vi "NI6602.ProcCases.vi"(0 "i ref in":refnum<vi>, 1 "selector":string, 2 "Data":T1, 3 "call cluster":T2={"Object"="", "Selector"="", "CallType"=enum."synchronous", "Async Object"="", "Async Selector"="", "Data Descriptor"="", "Data"=[], "Error #"=0, "Expire"=0}, 5 "error in (no error)":errorcluster) -> (14 "i ref out":refnum<vi>, 17 "answer cluster":T2={"Object"="", "Selector"="", "CallType"=enum."synchronous", "Async Object"="", "Async Selector"="", "Data Descriptor"="", "Data"=[], "Error #"=0, "Expire"=0}, 19 "error out":errorcluster)   [LabVIEW 2014, in "NI6602.lvlib"]
doc: "This method is called by a process from within the default case in the event loop. The methods of a class that are linked to events will be called from THIS method. Add your code here."
uses:
  NI6602.lvlib
  CS_Core/BaseProcess/BaseProcess.lvlib
  CS_Core/CSApplicationBaseClasses/DeviceBase/DeviceBase.lvlib
  CS_Core/CSSystem/CoreLib/CoreLib.string 2 byte array.vi
  CS_Core/CSSystem/CoreLib/CoreLib.lvlib
  CSlibraries-extern/DimLVEvent/LVDimInterface/LVDimInterface.lvlib
  CS_Core/CSSystem/CoreLib/CoreLib.byte array 2 double.vi
  CS_Core/CSSystem/CoreDefs/CoreDefs.call_type.ctl
  CS_Core/CSSystem/CoreDefs/CoreDefs.rawDataType.ctl
  CS_Core/BaseProcess/BaseProcess.descriptor string definition.ctl
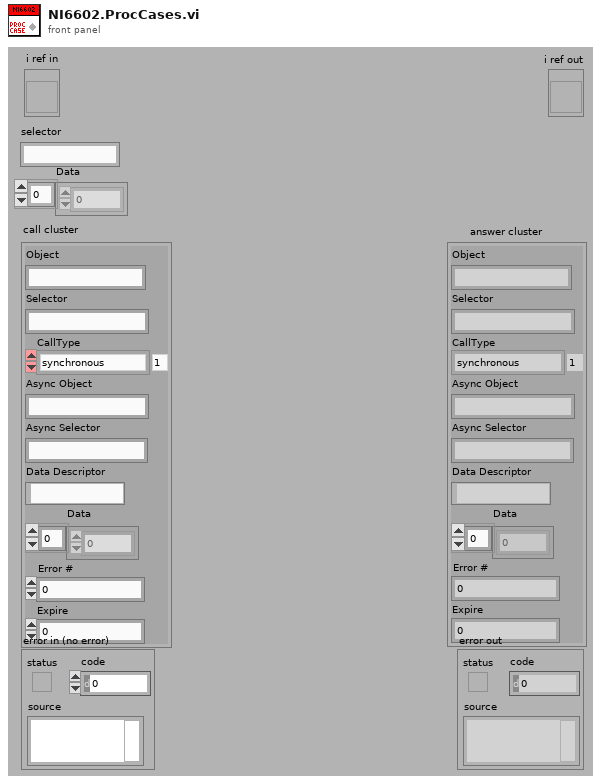
[diagram p1: front panel]
types:
  T1 = typedef "CoreDefs.rawDataType.ctl" = i8[]
  T2 = typedef "CoreDefs.call_type.ctl" = cluster{"Object":string, "Selector":string, "CallType":enum16{"simple", "synchronous", "asynchronous"}, "Async Object":string, "Async Selector":string, "Data Descriptor":T3, "Data":T1, "Error #":i32, "Expire":u32}
  T3 = typedef "BaseProcess.lvlib/BaseProcess.descriptor string definition.ctl" = string
  T4 = typedef "NI6602.lvlib/NI6602.i attribute.ctl" = cluster{"CounterDAQ Channels":cluster{"task":refnum<k21>, "Channel Name":string}[], "RateServiceIDs":i32[], "Running?":bool, "IntegralServiceIDs":i32[], "ThresholdID":i32, "Threshold":dbl, "IntegralValues":dbl[], "Stopped?":bool}
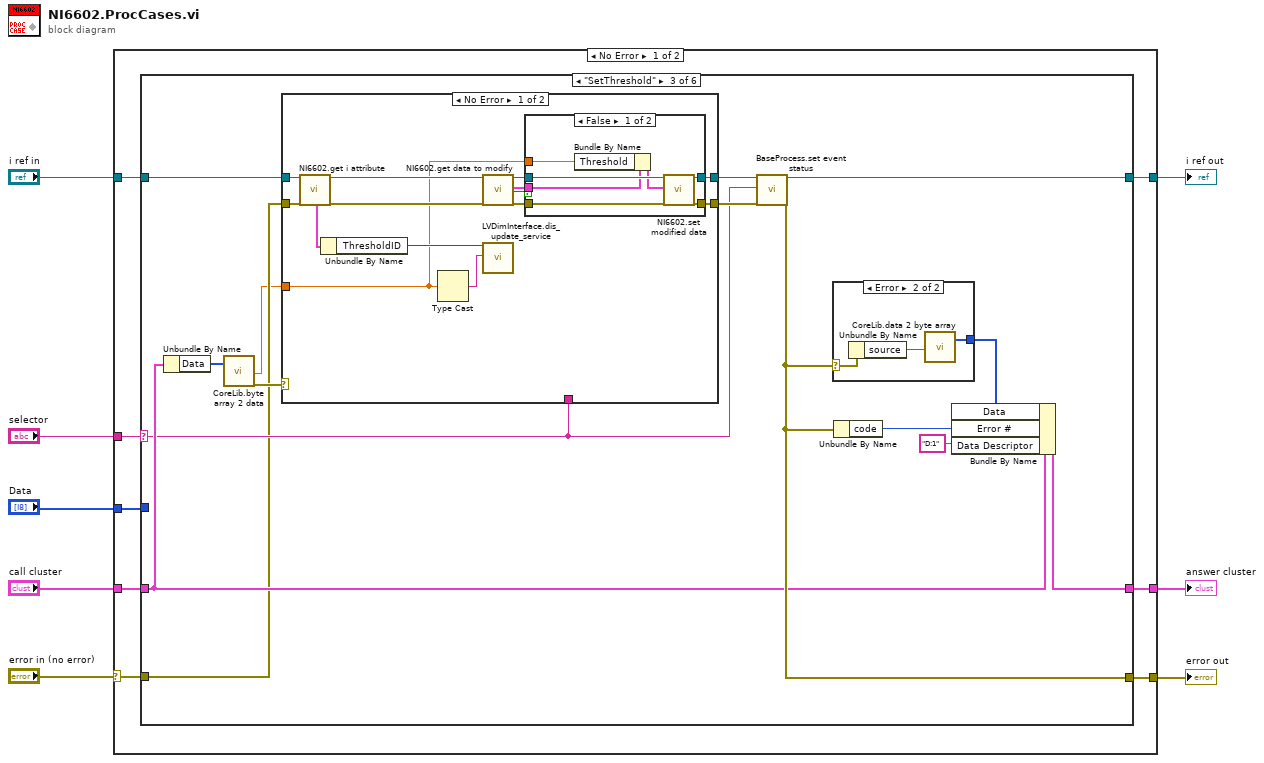
[diagram p0: block diagram]
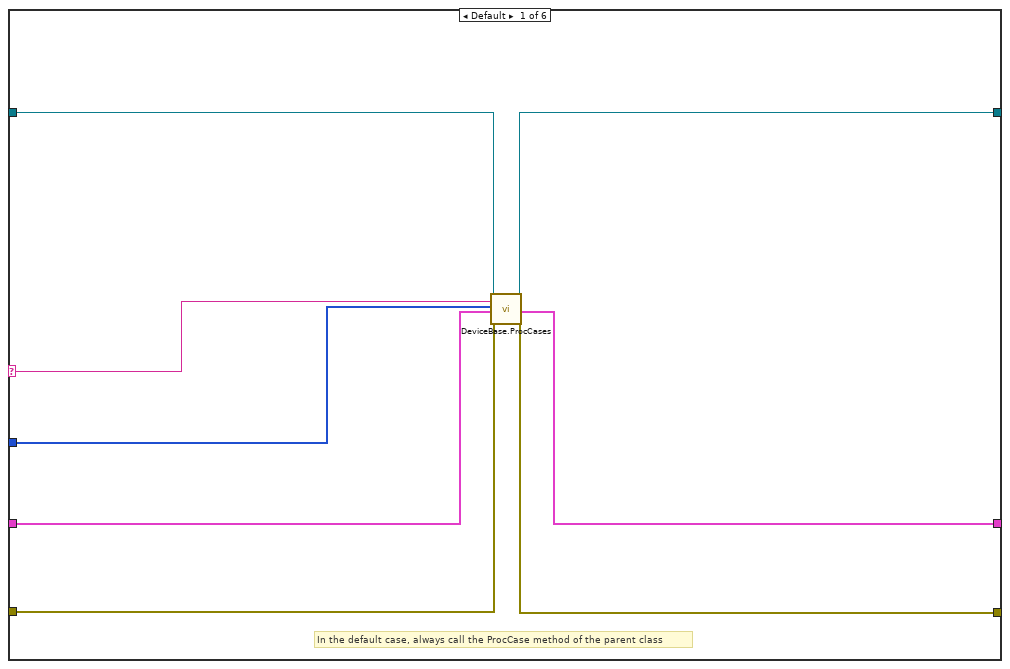
[diagram p2: hidden frame]
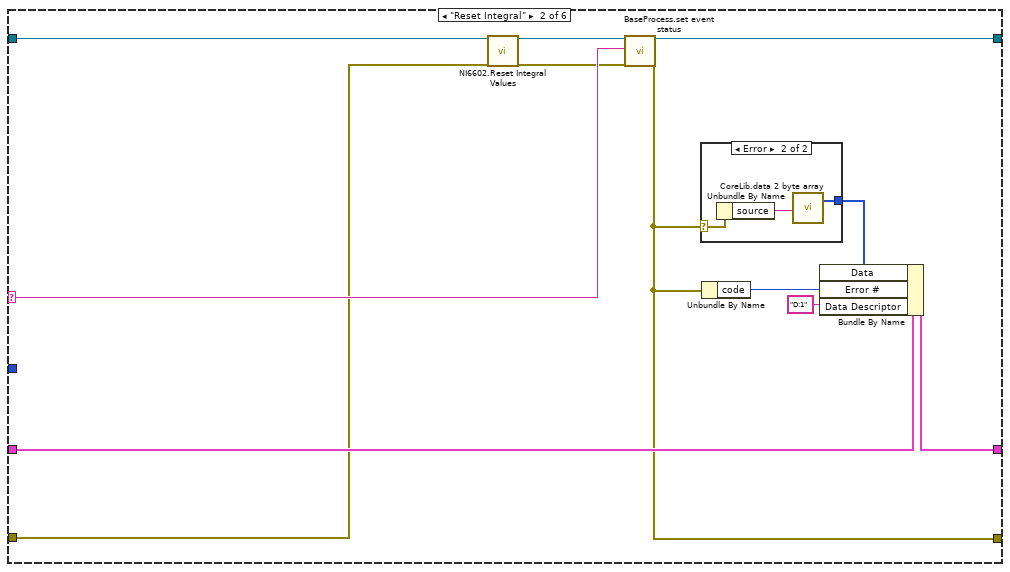
[diagram p3: hidden frame]
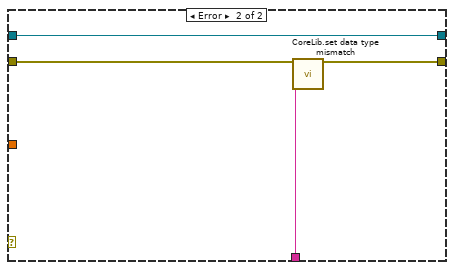
[diagram p6: hidden frame]
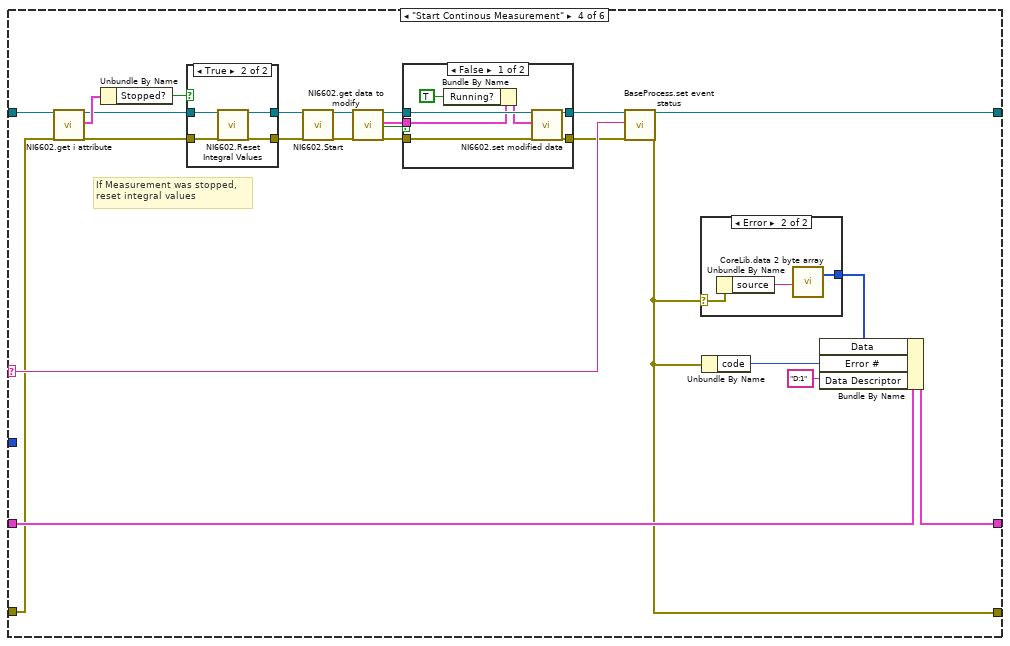
[diagram p8: hidden frame]
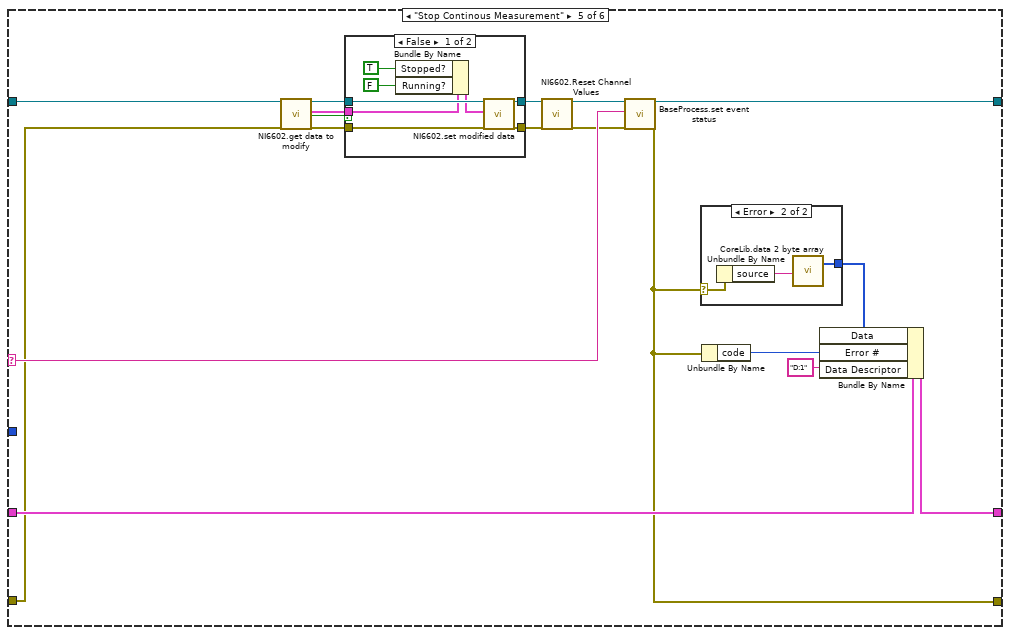
[diagram p12: hidden frame]
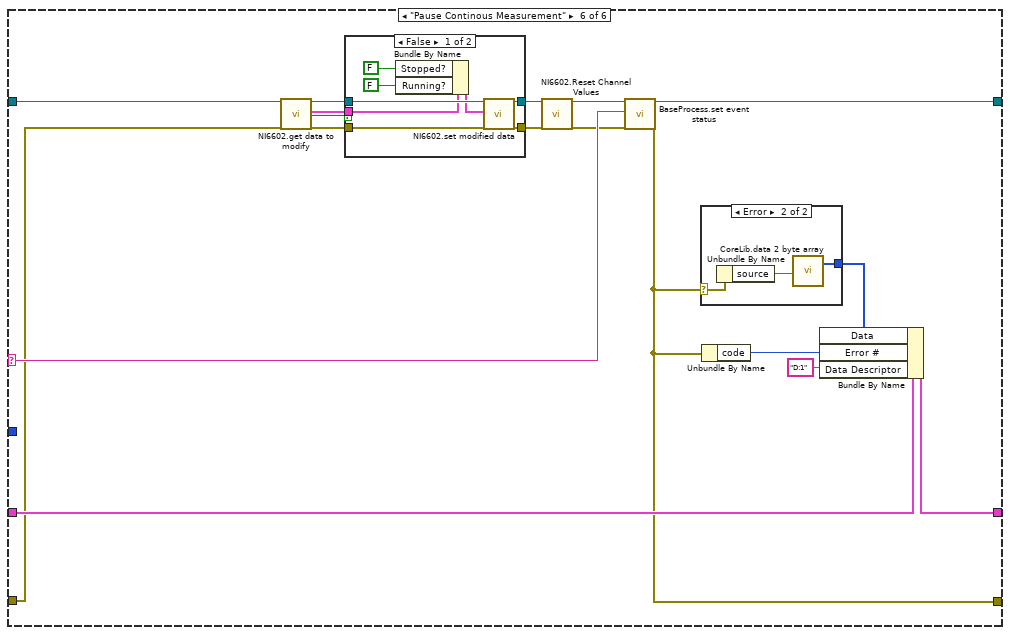
[diagram p15: hidden frame]
diagram:
  n1 = case shown="No Error" "error in (no error)" {
    selector: "error in (no error)" -> [w9 w189]
    tunnel: "selector" -> [w16 _]
    tunnel: [w15 w190] -> w7
    tunnel: "Data" -> [w14 _]
    tunnel: "call cluster" -> [w13 w190]
    tunnel: "i ref in" -> [w12 w191]
    tunnel: [w11 w191] -> w3
    tunnel: [w10 w189] -> w2
    frame No Error {
      n2 = case shown="\"SetThreshold\"" w16 {
        selector: w16 -> [w19 w31 w43 w103 w139 w170]
        tunnel: w14 -> [w17 _ _ _ _ _]
        tunnel: w12 -> [w18 w28 w40 w91 w131 w162]
        tunnel: [w24 w30 w50 w102 w138 w169] -> w11
        tunnel: w13 -> [w20 w35 w45 w107 w143 w174]
        tunnel: [w21 w34 w53 w106 w142 w173] -> w15
        tunnel: w9 -> [w23 w25 w42 w92 w132 w163]
        tunnel: [w22 w32 w51 w104 w140 w171] -> w10
        frame Default {
          # "In the default case, always call the ProcCase method of the parent class"
          n3 = call "DeviceBase.ProcCases.vi"("i ref in"=w18, "selector"=w19, "Data"=w17, "call cluster"=w20, "error in (no error)"=w23) -> ("i ref out"=w24:refnum<vi>, "answer cluster"=w21:T2, "error out"=w22:errorcluster)  [unwired: 12 in]
        }
        frame "Reset Integral" {
          n4 = call "NI6602.Reset Integral Values.vi"("i ref in"=w28, "error in (no error)"=w25) -> ("i ref out"=w27:refnum<vi>, "error out"=w26:errorcluster)  [unwired: 16 in]
          n5 = call "BaseProcess.set event status.vi"("i ref in"=w27, "EventStatus"=w31, "error in (no error)"=w26) -> ("i ref out"=w30:refnum<vi>, "error out"=w32:errorcluster)  [unwired: 14 in, 1 out]
          n6 = case shown="Error" w32 {
            selector: w32 -> [_ w39]
            tunnel: [_ w38] -> w33
            frame No Error {
            }
            frame Error {
              n7 = Unbundle By Name(w39) -> ("source"=w37:string)
              n8 = call-poly "CoreLib.data 2 byte array.vi"("string"=w37) -> ("byteArray out"=w38:T1)  [unwired: 18 in]
            }
          }
          n9 = Unbundle By Name(w32) -> ("code"=w36:i32)
          n10 = Bundle By Name(cluster=w35, "Data"=w33, "Error #"=w36, "Data Descriptor"="D:1") -> (w34:T2)
        }
        frame "SetThreshold" {
          n11 = Unbundle By Name(w45) -> ("Data"=w46:T1)
          n12 = call-poly "CoreLib.byte array 2 data.vi"("byteArray"=w46) -> ("d64"=w41:dbl, "error out"=w44:errorcluster)  [unwired: 16 in, 1 out]
          n13 = case shown="No Error" w44 {
            tunnel: [w64 w78] -> w48
            tunnel: [w63 w81] -> w47
            tunnel: w43 -> [_ w80]
            tunnel: w42 -> [w61 w79]
            tunnel: w41 -> [w55 _]
            tunnel: w40 -> [w60 w78]
            frame No Error {
              n14 = call "NI6602.get i attribute.vi"("i ref in"=w60, "error in (no error)"=w61) -> ("i ref out"=w59:refnum<vi>, "i attribute"=w58:T4, "error out"=w62:errorcluster)  [unwired: 15 in]
              n15 = Unbundle By Name(w58) -> ("ThresholdID"=w57:i32)
              n16 = Type Cast(x=w55) -> (*(type *) &x=w56:string)  [unwired: 1 in]
              n17 = call "NI6602.get data to modify.vi"("i ref in"=w59, "error in (no error)"=w62) -> ("i ref out"=w66:refnum<vi>, "i attribute"=w68:T4, "timed out"=w67:bool, "error out"=w65:errorcluster)  [unwired: 14 in]
              n18 = call "LVDimInterface.dis_update_service.vi"("my_serviceID"=w57, "data"=w56) -> ()  [unwired: 15 in, 3 out]
              n19 = case shown="False" w67 {
                tunnel: w65 -> [w75 w76]
                tunnel: [w74 w76] -> w63
                tunnel: w66 -> [w73 w77]
                tunnel: [w72 w77] -> w64
                tunnel: w68 -> [w71 _]
                tunnel: w55 -> [w69 _]
                frame False {
                  n20 = Bundle By Name(cluster=w71, "Threshold"=w69) -> (w70:T4)
                  n21 = call "NI6602.set modified data.vi"("i ref in"=w73, "i attribute"=w70, "error in (no error)"=w75) -> ("i ref out"=w72:refnum<vi>, "error out"=w74:errorcluster)  [unwired: 15 in]
                }
                frame True {
                }
              }
            }
            frame Error {
              n22 = call "CoreLib.set data type mismatch.vi"("error in (no error)"=w79, "error source"=w80) -> ("error out"=w81:errorcluster)  [unwired: 17 in]
            }
          }
          n23 = call "BaseProcess.set event status.vi"("i ref in"=w48, "EventStatus"=w43, "error in (no error)"=w47) -> ("i ref out"=w50:refnum<vi>, "error out"=w51:errorcluster)  [unwired: 14 in, 1 out]
          n24 = case shown="Error" w51 {
            selector: w51 -> [_ w84]
            tunnel: [_ w83] -> w52
            frame No Error {
            }
            frame Error {
              n25 = Unbundle By Name(w84) -> ("source"=w82:string)
              n26 = call-poly "CoreLib.data 2 byte array.vi"("string"=w82) -> ("byteArray out"=w83:T1)  [unwired: 18 in]
            }
          }
          n27 = Unbundle By Name(w51) -> ("code"=w54:i32)
          n28 = Bundle By Name(cluster=w45, "Data"=w52, "Error #"=w54, "Data Descriptor"="D:1") -> (w53:T2)
        }
        frame "Start Continous Measurement" {
          # "If Measurement was stopped,\nreset integral values"
          n29 = call "NI6602.get i attribute.vi"("i ref in"=w91, "error in (no error)"=w92) -> ("i ref out"=w87:refnum<vi>, "i attribute"=w90:T4, "error out"=w88:errorcluster)  [unwired: 15 in]
          n30 = Unbundle By Name(w90) -> ("Stopped?"=w89:bool)
          n31 = case shown="True" w89 {
            tunnel: w88 -> [w109 w114]
            tunnel: w87 -> [w110 w113]
            tunnel: [w110 w112] -> w86
            tunnel: [w109 w111] -> w85
            frame False {
            }
            frame True {
              n32 = call "NI6602.Reset Integral Values.vi"("i ref in"=w113, "error in (no error)"=w114) -> ("i ref out"=w112:refnum<vi>, "error out"=w111:errorcluster)  [unwired: 16 in]
            }
          }
          n33 = call "NI6602.Start.vi"("i ref in"=w86, "error in (no error)"=w85) -> ("i ref out"=w93:refnum<vi>, "error out"=w94:errorcluster)  [unwired: 16 in]
          n34 = call "NI6602.get data to modify.vi"("i ref in"=w93, "error in (no error)"=w94) -> ("i ref out"=w98:refnum<vi>, "i attribute"=w100:T4, "timed out"=w99:bool, "error out"=w97:errorcluster)  [unwired: 14 in]
          n35 = case shown="False" w99 {
            tunnel: w97 -> [w121 w122]
            tunnel: [w120 w122] -> w95
            tunnel: w98 -> [w119 w123]
            tunnel: [w118 w123] -> w96
            tunnel: w100 -> [w117 _]
            frame False {
              n36 = Bundle By Name(cluster=w117, "Running?"=TRUE) -> (w116:T4)
              n37 = call "NI6602.set modified data.vi"("i ref in"=w119, "i attribute"=w116, "error in (no error)"=w121) -> ("i ref out"=w118:refnum<vi>, "error out"=w120:errorcluster)  [unwired: 15 in]
            }
            frame True {
            }
          }
          n38 = call "BaseProcess.set event status.vi"("i ref in"=w96, "EventStatus"=w103, "error in (no error)"=w95) -> ("i ref out"=w102:refnum<vi>, "error out"=w104:errorcluster)  [unwired: 14 in, 1 out]
          n39 = case shown="Error" w104 {
            selector: w104 -> [_ w126]
            tunnel: [_ w125] -> w105
            frame No Error {
            }
            frame Error {
              n40 = Unbundle By Name(w126) -> ("source"=w124:string)
              n41 = call-poly "CoreLib.data 2 byte array.vi"("string"=w124) -> ("byteArray out"=w125:T1)  [unwired: 18 in]
            }
          }
          n42 = Unbundle By Name(w104) -> ("code"=w108:i32)
          n43 = Bundle By Name(cluster=w107, "Data"=w105, "Error #"=w108, "Data Descriptor"="D:1") -> (w106:T2)
        }
        frame "Stop Continous Measurement" {
          n44 = call "NI6602.get data to modify.vi"("i ref in"=w131, "error in (no error)"=w132) -> ("i ref out"=w134:refnum<vi>, "i attribute"=w136:T4, "timed out"=w135:bool, "error out"=w133:errorcluster)  [unwired: 14 in]
          n45 = case shown="False" w135 {
            tunnel: w133 -> [w152 w153]
            tunnel: [w151 w153] -> w130
            tunnel: w134 -> [w150 w154]
            tunnel: [w149 w154] -> w129
            tunnel: w136 -> [w148 _]
            frame False {
              n46 = Bundle By Name(cluster=w148, "Stopped?"=TRUE, "Running?"=FALSE) -> (w147:T4)
              n47 = call "NI6602.set modified data.vi"("i ref in"=w150, "i attribute"=w147, "error in (no error)"=w152) -> ("i ref out"=w149:refnum<vi>, "error out"=w151:errorcluster)  [unwired: 15 in]
            }
            frame True {
            }
          }
          n48 = call "NI6602.Reset Channel Values.vi"("i ref in"=w129, "error in (no error)"=w130) -> ("i ref out"=w127:refnum<vi>, "error out"=w128:errorcluster)  [unwired: 16 in]
          n49 = call "BaseProcess.set event status.vi"("i ref in"=w127, "EventStatus"=w139, "error in (no error)"=w128) -> ("i ref out"=w138:refnum<vi>, "error out"=w140:errorcluster)  [unwired: 14 in, 1 out]
          n50 = case shown="Error" w140 {
            selector: w140 -> [_ w157]
            tunnel: [_ w156] -> w141
            frame No Error {
            }
            frame Error {
              n51 = Unbundle By Name(w157) -> ("source"=w155:string)
              n52 = call-poly "CoreLib.data 2 byte array.vi"("string"=w155) -> ("byteArray out"=w156:T1)  [unwired: 18 in]
            }
          }
          n53 = Unbundle By Name(w140) -> ("code"=w144:i32)
          n54 = Bundle By Name(cluster=w143, "Data"=w141, "Error #"=w144, "Data Descriptor"="D:1") -> (w142:T2)
        }
        frame "Pause Continous Measurement" {
          n55 = call "NI6602.get data to modify.vi"("i ref in"=w162, "error in (no error)"=w163) -> ("i ref out"=w165:refnum<vi>, "i attribute"=w167:T4, "timed out"=w166:bool, "error out"=w164:errorcluster)  [unwired: 14 in]
          n56 = case shown="False" w166 {
            tunnel: w164 -> [w183 w184]
            tunnel: [w182 w184] -> w161
            tunnel: w165 -> [w181 w185]
            tunnel: [w180 w185] -> w160
            tunnel: w167 -> [w179 _]
            frame False {
              n57 = Bundle By Name(cluster=w179, "Stopped?"=FALSE, "Running?"=FALSE) -> (w178:T4)
              n58 = call "NI6602.set modified data.vi"("i ref in"=w181, "i attribute"=w178, "error in (no error)"=w183) -> ("i ref out"=w180:refnum<vi>, "error out"=w182:errorcluster)  [unwired: 15 in]
            }
            frame True {
            }
          }
          n59 = call "NI6602.Reset Channel Values.vi"("i ref in"=w160, "error in (no error)"=w161) -> ("i ref out"=w158:refnum<vi>, "error out"=w159:errorcluster)  [unwired: 16 in]
          n60 = call "BaseProcess.set event status.vi"("i ref in"=w158, "EventStatus"=w170, "error in (no error)"=w159) -> ("i ref out"=w169:refnum<vi>, "error out"=w171:errorcluster)  [unwired: 14 in, 1 out]
          n61 = case shown="Error" w171 {
            selector: w171 -> [_ w188]
            tunnel: [_ w187] -> w172
            frame No Error {
            }
            frame Error {
              n62 = Unbundle By Name(w188) -> ("source"=w186:string)
              n63 = call-poly "CoreLib.data 2 byte array.vi"("string"=w186) -> ("byteArray out"=w187:T1)  [unwired: 18 in]
            }
          }
          n64 = Unbundle By Name(w171) -> ("code"=w175:i32)
          n65 = Bundle By Name(cluster=w174, "Data"=w172, "Error #"=w175, "Data Descriptor"="D:1") -> (w173:T2)
        }
      }
    }
    frame Error {
    }
  }
  "answer cluster" <- w7
  "i ref out" <- w3
  "error out" <- w2
